vi "ExSpecAppCamera.vi"() -> ()   [LabVIEW 2010]
uses:
  GlobalSpectHdl.vi
  GlobalCamOpen.vi
  GlobalInitializeFlag.vi
  GlobalFramesToStr.vi
  GlobalTimingMode.vi
  GlobalAcquireFocusFlag.vi
  GlobalExposure.vi
  GlobalUserBin.vi
  GlobalCenter.vi
  GlobalFullBin.vi
  GlobalFlipFlag.vi
  GlobalReverseFlag.vi
  GlobalIBackImgHndl.vi
  GlobalIFlatImgHndl.vi
panel:
  out "Spectrometer Active":bool
  in  "Select Spectrometer":bool
  out "Camera Opened":bool
  in  "Exit program":bool
  out "error out":errorcluster
  in  "error in (no error)":errorcluster
  in  "Tab Control":T1(tab)
  in  "Focus/Acquire Mode":u32=1 min=1 max=5 step=1
  in  "Number of Frames to store":u32=1 min=1 step=1
  in  "Intensifier":bool
  in  "Readout Port":i32=-1 min=-1 step=1
  in  "ADC Offset 2":i32=-1 min=-1 step=1
  in  "ADC Gain 2":i32=-1 min=-1 step=1
  in  "ADC speed":i32=-2 min=-3 step=1
  in  "Trigger Edge":u32(ring)=1 items=["N/A", "Positive (leading) edge", "Negative (falling) edge"]
  in  "Timing Mode":u32(ring)=1 items=["N/A", "Free Run/Timed", "Trigger First (PM only)", "Ext Sync/Strobed ", "Variable Exp (PM only)", "Flash Mode (PM only)"]
  out "Pixel Time":i32
  out "Bit Depth":i32
  out "ReadOut port":i32
  out "ADC Offset":i32
  out "ADC Gain":i32
  out "ADC Speed":i32
  in  "Set Experiment \nParameters, Initialize \nCamera/Controller":bool
  out "temperature":dbl format="%.2f"
  out "Temperature Read":dbl(slide) scale=-120.0..20.0
  in  "Temperature":dbl format="%.2f"
  in  "Exposure":dbl format="%.2f"
  out "Controller Initialized":bool
  out "Total":u32
  out "Y dim":u32
  out "X dim":u32
  in  "Y Bin":u32=1 min=1 step=1
  in  "Y Start":u32=1 min=1 step=1
  out "center":bool
  out "User":bool
  out "Full":bool
  in  "Center Strip Button":bool
  in  "User Defined Button":bool
  in  "Full strip Button":bool
  out "Flip\nActive":bool
  in  "Flip flag Button":bool
  out "Reverse\nActive":bool
  in  "Image Reverse Button":bool
  out "Flat Field\nActive":bool
  out "Background \nActive":bool
  in  "Frame number to read":u32=1 min=1 step=1
  in  "Flat Button":bool
  in  "Back Button":bool
  in  "Full File Name":path
  in  "FileType":u32=67371008
  in  "Get Spectrometer \nInformation":bool
  in  "Set Spectrometer":bool
  out "Current Speed":dbl format="%.2f"
  out "Current Gratting":u32
  out "Current Wavelength":dbl format="%.2f"
  in  "Grating number":u32=1 min=1 step=1
  in  "Wavelength":dbl format="%.2f"
  out "Focus graph":sgl[](graph)
  out "Reverse active":bool
  out "Flat Field active":bool
  out "Background active":bool
  in  "Reverse\nbutton":bool
  in  "Flat Field\nbutton":bool
  in  "Background\nbutton":bool
  in  "stop 2":bool
  in  "Start":bool
  out "Camera initialized":bool
  out "Acquire Graph":sgl[](graph)
  out "Collecting Data":bool
  in  "Full File Name for Acqure":path
  in  "OK Button":bool
  out "camera initialized":bool
  # "Note: In order for any parameters to change and be downloaded the initialize button must be hit."
  # "The following are read \nfrom camera after setting\nvalues to left.\n-1 value means item is not \nsupported by camera."
  # "For Slowest ADC speed set this to -3\nFor Fastest ADC speed set this to -2\nTo use current ADC speed don't  hook up or use -1\notherwise put speed in as kHz"
  # "To use current gain don't hook up or set to -1"
  # "To use current gain don't hook up or set to -1"
  # "To use current gain don't hook up or set to -1"
  # "NOTE: if you are using background subtraction or flat field and you change \nthe ROI there are no checks in this example for this."
  # "Pixels coming back\nfrom Camera"
  # "File Types:\nSPE = 67371008\nTIF   = 67174400\nPMI  = 67436544"
  # "Browse match pattern is set to *.tif.  Modify this if different file type is needed."
  # "Note: This is an example only, the user has to verify that the x,y dimensions match for \nthe background and flat field files with the ROI. This error checking logic is not in this \nexample."
  # "Instructions:\nMake sure camera/controller has been initialized, led should be on.\nPress start button, display should appear.\nWhen done press stop button, display should disappear.\nLive buttons only work while collecting data, not before, to setup before goto Live operations tab."
  # "Online operations, will only work while collecting data."
  # "Be sure to put in a full file name below before starting."
  # "Instructions:\nMake sure the camera/controller has been initialized, the light should be on.\nMake sure to put in a file name with path to save data.\nPress Start button and display will pop up and data well be saved in file."
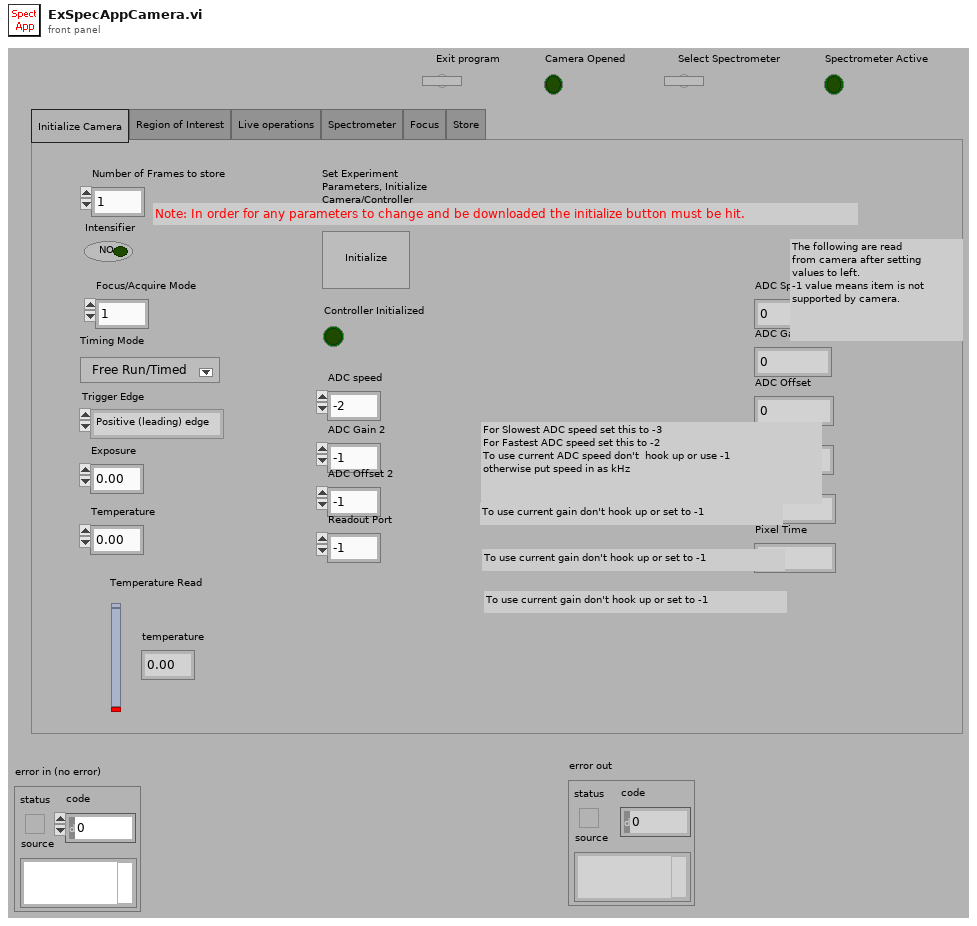
[diagram p1: front panel]
types:
  T1 = enum32{"Initialize Camera", "Region of Interest", "Live operations", "Spectrometer", "Focus", "Store"}
  T2 = cluster{"Camera Handle":u32, "Pulser Handle":u32, "File Handle":u32, "Display Handle":u32, "Image Handle":u32}
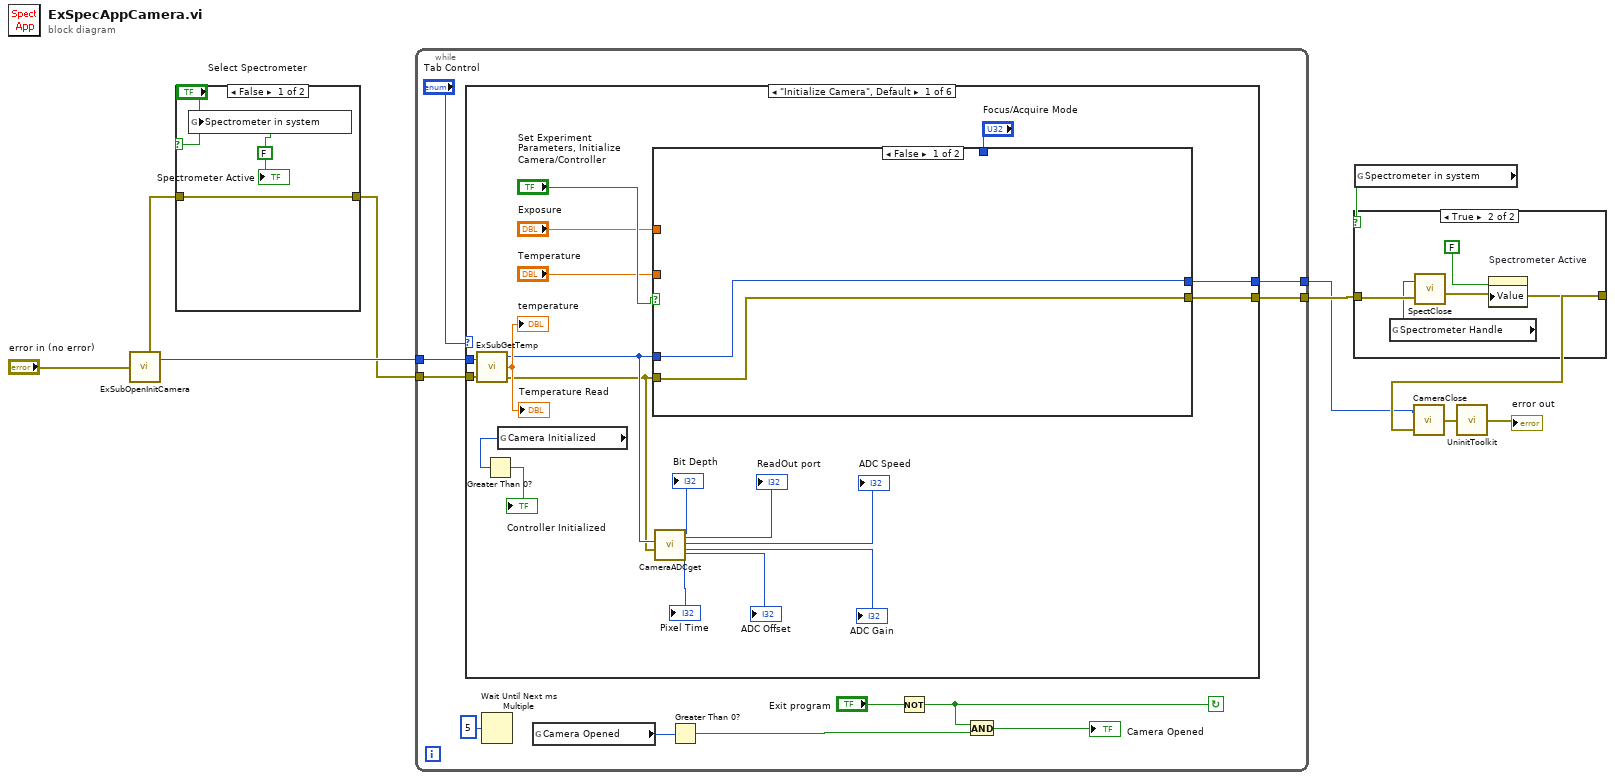
[diagram p0: block diagram]
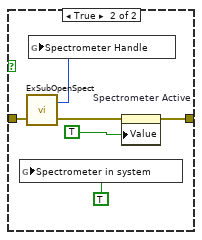
[diagram p3: hidden frame]
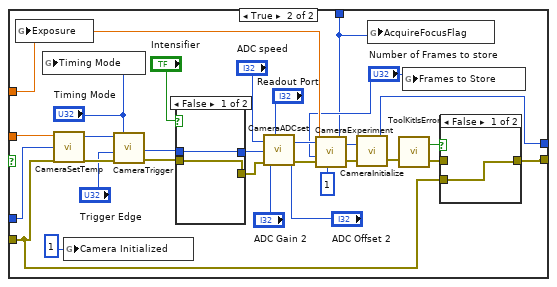
[diagram p4: hidden frame]
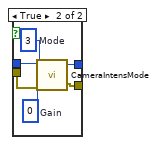
[diagram p6: hidden frame]
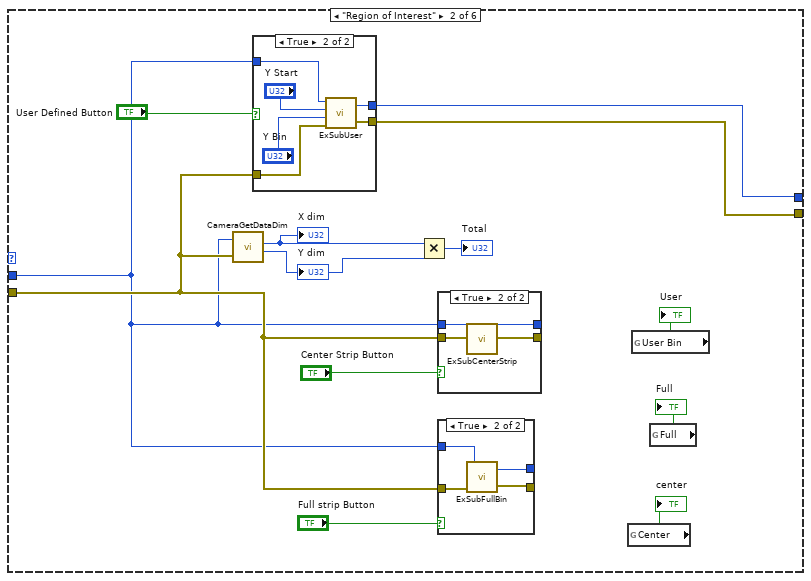
[diagram p7: hidden frame]
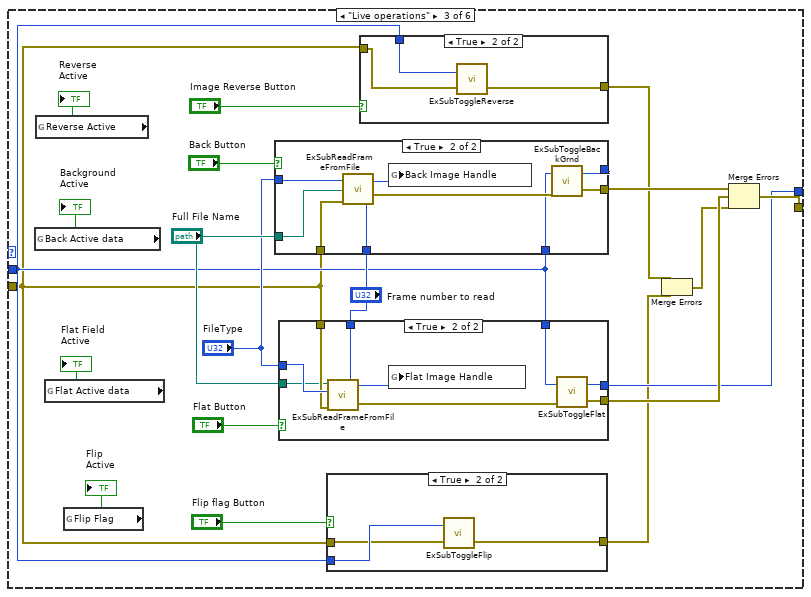
[diagram p11: hidden frame]
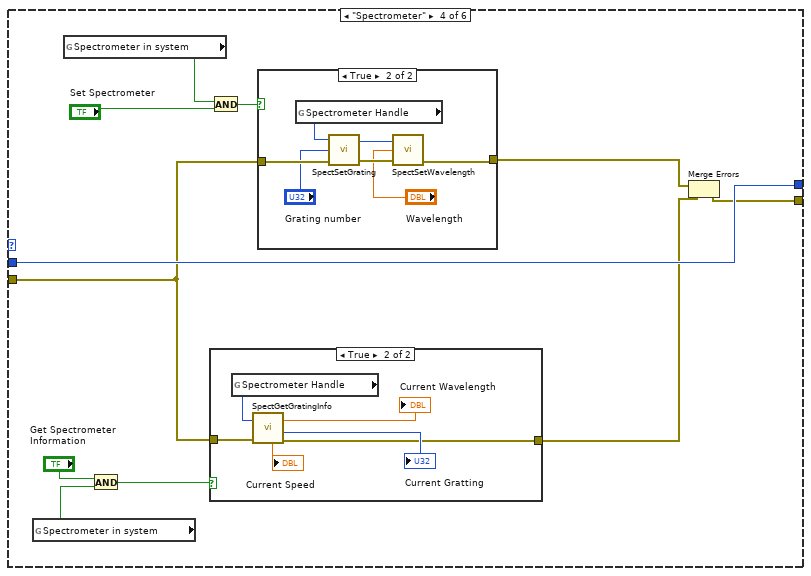
[diagram p16: hidden frame]
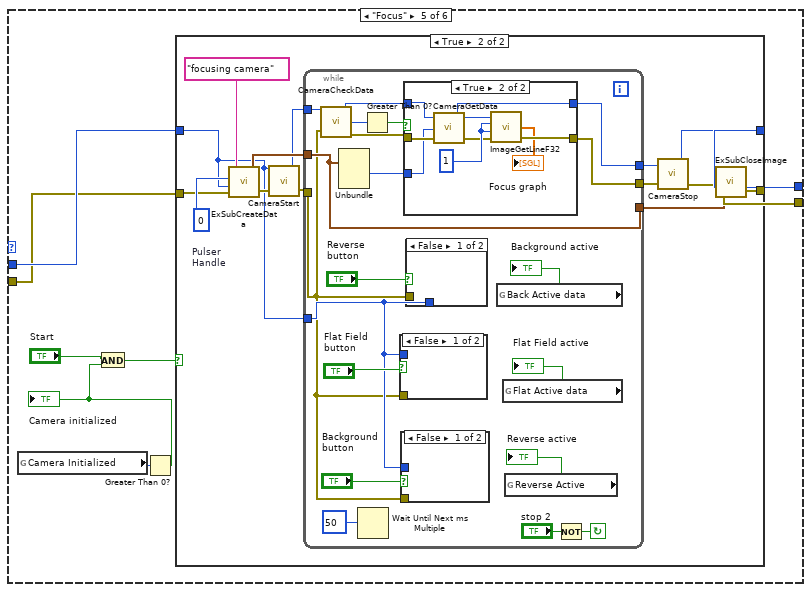
[diagram p19: hidden frame]
diagram:
  n1 = call "ExSubOpenInitCamera.vi"("error in (no error)"="error in (no error)") -> ("Camera Handle"=w2:u32, "error out"=w3:errorcluster)
  n2 = case shown="False" "Select Spectrometer" {
    tunnel: w3 -> [w12 w18]
    tunnel: [w12 w15] -> w1
    frame False {
      w13 = FALSE
      n3 = global write "GlobalSpectHdl.vi" "Spectrometer in system"(w13) -> ()
      "Spectrometer Active" <- w13
    }
    frame True {
      n4 = global write "GlobalSpectHdl.vi" "Spectrometer in system"(TRUE) -> ()
      n5 = call "ExSubOpenSpect.vi"("error in (no error)"=w18) -> ("Spectromete Handle"=w14:u32, "error out"=w17:errorcluster)
      n6 = global write "GlobalSpectHdl.vi" "Spectrometer Handle"(w14) -> ()
      n7 = property on="Spectrometer Active" class="Bool (strict)"(error in=w17, "Value"=TRUE) -> (error out=w15:errorcluster)  [unwired: 1 in, 1 out]
    }
  }
  n8 = while {
    tunnel: w2 -> [w30]
    tunnel: w1 -> [w27]
    tunnel: [w26] -> w6
    tunnel: [w25] -> w8
    stop <- w23 continue-if-true
    n9 = case shown="\"Initialize Camera\", Default" "Tab Control" {
      tunnel: w30 -> [w49 w98 w129 w185 w202 w266]
      tunnel: w27 -> [w41 w99 w128 w178 w201 w265]
      tunnel: [w33 w97 w136 w185 w204 w263] -> w26
      tunnel: [w32 w96 w137 w177 w203 w264] -> w25
      frame "Initialize Camera", Default {
        n10 = call "ExSubGetTemp.vi"("Camera Handle"=w49, "error in (no error)"=w41) -> ("Camera Handle"=w40:u32, "Temperature Real"=→"temperature" →"Temperature Read":dbl, "error out"=w39:errorcluster)
        n11 = global read "GlobalInitializeFlag.vi" "Camera Initialized"() -> (w44:u32)
        n12 = Greater Than 0?(x=w44) -> (x > 0?=→"Controller Initialized":bool)
        n13 = case shown="False" "Set Experiment \nParameters, Initialize \nCamera/Controller" {
          tunnel: "Exposure" -> [_ w70]
          tunnel: "Temperature" -> [_ w79]
          tunnel: w39 -> [w50 w54]
          tunnel: w40 -> [w51 w80]
          tunnel: [w50 w57] -> w32
          tunnel: [w51 w55] -> w33
          tunnel: "Focus/Acquire Mode" -> [_ w52]
          frame False {
          }
          frame True {
            n14 = global write "GlobalExposure.vi" "Exposure"(w70) -> ()
            n15 = global write "GlobalTimingMode.vi" "Timing Mode"("Timing Mode") -> ()
            n16 = call <userlib>:"CameraSetTemp.vi"("error in (no error)"=w54, "Temperature"=w79, "Camera Handle"=w80) -> ("error out"=w69:errorcluster, "Camera Handle"=w68:u32)
            n17 = global write "GlobalInitializeFlag.vi" "Camera Initialized"(1) -> ()
            n18 = call <userlib>:"CameraTrigger.vi"("error in"=w69, "Trigger Edge"="Trigger Edge", "Timing Mode"="Timing Mode", "Camera Handle"=w68) -> ("error out"=w65:errorcluster, "Camera Handle"=w66:u32)
            n19 = case shown="False" "Intensifier" {
              tunnel: [w85 w91] -> w76
              tunnel: [w84 w90] -> w77
              tunnel: w66 -> [w85 w87]
              tunnel: w65 -> [w84 w86]
              frame False {
              }
              frame True {
                w88 = u32 0  # Gain
                w89 = u32 3  # Mode
                n20 = call <userlib>:"CameraIntensMode.vi"("error in"=w86, "Intensifier Gain"=w88, "Mode"=w89, "Camera Handle"=w87) -> ("error out"=w90:errorcluster, "Camera Handle"=w91:u32)
              }
            }
            n21 = call <userlib>:"CameraADCset.vi"("ADC offset"="ADC Offset 2", "Read Out port"="Readout Port", "error in (no error)"=w77, "ADC Gain"="ADC Gain 2", "ADC Speed"="ADC speed", "Camera Handle"=w76) -> ("error out"=w63:errorcluster, "Camera Handle"=w62:u32)
            n22 = call <userlib>:"CameraExperiment.vi"("Number of Accumulations"=1, "Acquire / Focus Flag"=w52, "error in"=w63, "Number of Images"="Number of Frames to store", "Exposure (sec)"=w70, "Camera Handle"=w62) -> ("error out"=w61:errorcluster, "Camera Handle"=w60:u32)
            n23 = call <userlib>:"CameraInitialize.vi"("error in"=w61, "Camera Handle"=w60) -> ("error out"=w56:errorcluster, "Camera Handle"=w55:u32)
            n24 = global write "GlobalAcquireFocusFlag.vi" "AcquireFocusFlag"(w52) -> ()
            n25 = call <userlib>:"ToolKitIsError.vi"("error in"=w56) -> ("error out"=w58:errorcluster, "Error Flag"=w59:bool)  [unwired: 1 in]
            n26 = global write "GlobalFramesToStr.vi" "Frames to Store"("Number of Frames to store") -> ()
            n27 = case shown="False" w59 {
              tunnel: w58 -> [_ w83]
              tunnel: [w82 w83] -> w57
              tunnel: w54 -> [w82 _]
              frame False {
              }
              frame True {
              }
            }
          }
        }
        n28 = call <userlib>:"CameraADCget.vi"("Camera handle"=w40, "error in (no error)"=w39) -> ("Bit Depth"=→"Bit Depth":i32, "Pixel Time"=→"Pixel Time":i32, "Readout Port"=→"ReadOut port":i32, "ADC Offset"=→"ADC Offset":i32, "ADC Speed"=→"ADC Speed":i32, "ADC Gain"=→"ADC Gain":i32)  [unwired: 2 out]
      }
      frame "Region of Interest" {
        n29 = call <userlib>:"CameraGetDataDim.vi"("Camera Handle"=w98, "error in"=w99) -> ("Xdim"=w95:u32, "Ydim"=w94:u32)  [unwired: 2 out]
        "X dim" <- w95
        "Y dim" <- w94
        n30 = case shown="True" "User Defined Button" {
          tunnel: w98 -> [w117 w124]
          tunnel: [w117 w119] -> w97
          tunnel: w99 -> [w118 w121]
          tunnel: [w118 w120] -> w96
          frame False {
          }
          frame True {
            n31 = call "ExSubUser.vi"("error in (no error)"=w121, "Y Bin"="Y Bin", "Y Start"="Y Start", "Camera Handle"=w124) -> ("error out"=w120:errorcluster, "Camera Handle"=w119:u32)
          }
        }
        n32 = Multiply(x=w95, y=w94) -> (x*y=→"Total":u32)
        n33 = case shown="True" "Center Strip Button" {
          tunnel: w98 -> [w112 w115]
          tunnel: [w112 w114] -> _
          tunnel: w99 -> [w111 w116]
          tunnel: [w111 w113] -> _
          frame False {
          }
          frame True {
            n34 = call "ExSubCenterStrip.vi"("error in (no error)"=w116, "Camera Handle"=w115) -> ("error out"=w113:errorcluster, "Camera Handle"=w114:u32)
          }
        }
        n35 = case shown="True" "Full strip Button" {
          tunnel: w98 -> [w106 w110]
          tunnel: [w106 w108] -> _
          tunnel: w99 -> [w105 w109]
          tunnel: [w105 w107] -> _
          frame False {
          }
          frame True {
            n36 = call "ExSubFullBin.vi"("error in (no error)"=w109, "Camera Handle"=w110) -> ("error out"=w107:errorcluster, "Camera Handle"=w108:u32)
          }
        }
        n37 = global read "GlobalCenter.vi" "Center"() -> (→"center":bool)
        n38 = global read "GlobalUserBin.vi" "User Bin"() -> (→"User":bool)
        n39 = global read "GlobalFullBin.vi" "Full"() -> (→"Full":bool)
      }
      frame "Live operations" {
        n40 = global read "GlobalIBackImgHndl.vi" "Back Active data"() -> (→"Background \nActive":bool)
        n41 = global read "GlobalReverseFlag.vi" "Reverse Active"() -> (→"Reverse\nActive":bool)
        n42 = global read "GlobalIFlatImgHndl.vi" "Flat Active data"() -> (→"Flat Field\nActive":bool)
        n43 = global read "GlobalFlipFlag.vi" "Flip Flag"() -> (→"Flip\nActive":bool)
        n44 = case shown="True" "Back Button" {
          tunnel: "Full File Name" -> [_ w172]
          tunnel: "FileType" -> [_ w173]
          tunnel: w128 -> [w165 w174]
          tunnel: [w165 w168] -> w139
          tunnel: "Frame number to read" -> [_ w171]
          tunnel: w129 -> [w164 w167]
          tunnel: [w164 w166] -> _
          frame False {
          }
          frame True {
            n45 = call "ExSubReadFrameFromFile.vi"("error in (no error)"=w174, "Frame to pull off"=w171, "File type"=w173, "path to file to open"=w172) -> ("error out"=w169:errorcluster, "Image Handle"=w170:u32)
            n46 = global write "GlobalIBackImgHndl.vi" "Back Image Handle"(w170) -> ()
            n47 = call "ExSubToggleBackGrnd.vi"("error in (no error)"=w169, "Camera Handle"=w167) -> ("error out"=w168:errorcluster, "Camera Handle"=w166:u32)
          }
        }
        n48 = case shown="True" "Flat Button" {
          tunnel: "Full File Name" -> [_ w160]
          tunnel: "FileType" -> [_ w163]
          tunnel: w128 -> [w154 w161]
          tunnel: [w154 w156] -> w138
          tunnel: "Frame number to read" -> [_ w162]
          tunnel: w129 -> [w153 w158]
          tunnel: [w153 w157] -> w136
          frame False {
          }
          frame True {
            n49 = call "ExSubReadFrameFromFile.vi"("error in (no error)"=w161, "Frame to pull off"=w162, "File type"=w163, "path to file to open"=w160) -> ("error out"=w155:errorcluster, "Image Handle"=w159:u32)
            n50 = global write "GlobalIFlatImgHndl.vi" "Flat Image Handle"(w159) -> ()
            n51 = call "ExSubToggleFlat.vi"("error in (no error)"=w155, "Camera Handle"=w158) -> ("error out"=w156:errorcluster, "Camera Handle"=w157:u32)
          }
        }
        n52 = case shown="True" "Flip flag Button" {
          tunnel: w129 -> [_ w152]
          tunnel: w128 -> [w149 w151]
          tunnel: [w149 w150] -> w127
          frame False {
          }
          frame True {
            n53 = call "ExSubToggleFlip.vi"("error in (no error)"=w151, "Camera Handle"=w152) -> ("error out"=w150:errorcluster)  [unwired: 1 out]
          }
        }
        n54 = case shown="True" "Image Reverse Button" {
          tunnel: w129 -> [_ w147]
          tunnel: w128 -> [w145 w148]
          tunnel: [w145 w146] -> w126
          frame False {
          }
          frame True {
            n55 = call "ExSubToggleReverse.vi"("error in (no error)"=w148, "Camera Handle"=w147) -> ("error out"=w146:errorcluster)  [unwired: 1 out]
          }
        }
        n56 = Merge Errors(w126, w127) -> (w125:errorcluster)
        n57 = Merge Errors(w139, w138, w125) -> (w137:errorcluster)
      }
      frame "Spectrometer" {
        n58 = global read "GlobalSpectHdl.vi" "Spectrometer in system"() -> (w181:bool)
        n59 = global read "GlobalSpectHdl.vi" "Spectrometer in system"() -> (w184:bool)
        n60 = And(x="Get Spectrometer \nInformation", y=w181) -> (x .and. y?=w179:bool)
        n61 = case shown="True" w179 {
          tunnel: w178 -> [w186 w191]
          tunnel: [w186 w188] -> w176
          frame False {
          }
          frame True {
            n62 = global read "GlobalSpectHdl.vi" "Spectrometer Handle"() -> (w192:u32)
            n63 = call <userlib>:"SpectGetGratingInfo.vi"("Spectrometer Handle"=w192, "error in"=w191) -> ("Current Wavelength"=→"Current Wavelength":dbl, "Current Speed"=→"Current Speed":dbl, "Current Grating"=→"Current Gratting":i16, "error out"=w188:errorcluster)  [unwired: 2 out]
          }
        }
        n64 = And(x=w184, y="Set Spectrometer") -> (x .and. y?=w182:bool)
        n65 = case shown="True" w182 {
          tunnel: w178 -> [w193 w199]
          tunnel: [w193 w194] -> w175
          frame False {
          }
          frame True {
            n66 = global read "GlobalSpectHdl.vi" "Spectrometer Handle"() -> (w200:u32)
            n67 = call <userlib>:"SpectSetGrating.vi"("error in"=w199, "Grating Number"="Grating number", "Sepctrometer Handle"=w200) -> ("error out"=w196:errorcluster, "Spectrometer Handle"=w197:u32)
            n68 = call <userlib>:"SpectSetWavelength.vi"("error in"=w196, "Wavelength"="Wavelength", "Spectrometer Handle"=w197) -> ("error out"=w194:errorcluster)  [unwired: 1 out]
          }
        }
        n69 = Merge Errors(w175, w176) -> (w177:errorcluster)
      }
      frame "Focus" {
        n70 = global read "GlobalInitializeFlag.vi" "Camera Initialized"() -> (w206:u32)
        n71 = Greater Than 0?(x=w206) -> (x > 0?=w205:bool)
        "Camera initialized" <- w205
        n72 = And(x="Start", y=w205) -> (x .and. y?=w208:bool)
        n73 = case shown="True" w208 {
          tunnel: w201 -> [w209 w220]
          tunnel: w202 -> [w210 w213]
          tunnel: [w210 w218] -> w204
          tunnel: [w209 w217] -> w203
          frame False {
          }
          frame True {
            w221 = u32 0  # Pulser  Handle
            n74 = call "ExSubCreateData.vi"("error in (no error)"=w220, "File and Display Name"="focusing camera", "Pulser Handle"=w221, "Camera Handle"=w213) -> ("error out"=w222:errorcluster, "Handles Out"=w224:T2)
            n75 = call <userlib>:"CameraStart.vi"("error in"=w222, "Camera Handle"=w213) -> ("error out"=w223:errorcluster, "Camera Handle"=w215:u32)
            n76 = while {
              tunnel: w224 -> [w226]
              tunnel: w223 -> [w225]
              tunnel: w213 -> [w238]
              tunnel: w215 -> [w230]
              tunnel: [w229] -> w214
              tunnel: [w228] -> w212
              tunnel: [w226] -> w211
              stop <- w242 continue-if-true
              n77 = call <userlib>:"CameraCheckData.vi"("Camera Handle"=w230, "error in"=w225) -> ("Camera Handle"=w232:u32, "Number Of Frames Available"=w234:i32, "error out"=w231:errorcluster)
              n78 = Unbundle(w226) -> ("Image Handle"=w227:u32)  [unwired: 4 out]
              n79 = Wait Until Next ms Multiple(millisecond multiple=u32 50) -> ()  [unwired: 1 out]
              n80 = Greater Than 0?(x=w234) -> (x > 0?=w233:bool)
              n81 = case shown="False" "Flat Field\nbutton" {
                tunnel: w238 -> [_ w258]
                tunnel: w225 -> [_ w259]
                frame False {
                }
                frame True {
                  n82 = call "ExSubToggleFlat.vi"("error in (no error)"=w259, "Camera Handle"=w258) -> ()  [unwired: 2 out]
                }
              }
              n83 = case shown="False" "Background\nbutton" {
                tunnel: w238 -> [_ w257]
                tunnel: w225 -> [_ w256]
                frame False {
                }
                frame True {
                  n84 = call "ExSubToggleBackGrnd.vi"("error in (no error)"=w256, "Camera Handle"=w257) -> ()  [unwired: 2 out]
                }
              }
              n85 = case shown="True" w233 {
                tunnel: w232 -> [w246 w255]
                tunnel: w231 -> [w245 w254]
                tunnel: [w245 w249] -> w228
                tunnel: [w246 w248] -> w229
                tunnel: w227 -> [_ w253]
                frame False {
                }
                frame True {
                  w251 = 1
                  n86 = call <userlib>:"CameraGetData.vi"("error in"=w254, "Data Handle"=w253, "Camera Handle"=w255) -> ("error out"=w250:errorcluster, "Data Handle"=w252:u32, "Camera Handle"=w248:u32)
                  n87 = call <userlib>:"ImageGetLineF32.vi"("error in"=w250, "Z Position"=w251, "Y Position"=w251, "Data Handle"=w252) -> ("error out"=w249:errorcluster, "Array F32"=→"Focus graph":sgl[])  [unwired: 1 out]
                }
              }
              n88 = case shown="False" "Reverse\nbutton" {
                tunnel: w225 -> [_ w261]
                tunnel: w238 -> [_ w260]
                frame False {
                }
                frame True {
                  n89 = call "ExSubToggleReverse.vi"("error in (no error)"=w261, "Camera Handle"=w260) -> ()  [unwired: 2 out]
                }
              }
              n90 = global read "GlobalIBackImgHndl.vi" "Back Active data"() -> (→"Background active":bool)
              n91 = global read "GlobalIFlatImgHndl.vi" "Flat Active data"() -> (→"Flat Field active":bool)
              n92 = global read "GlobalReverseFlag.vi" "Reverse Active"() -> (→"Reverse active":bool)
              n93 = Not(x="stop 2") -> (.not. x?=w242:bool)
            }
            n94 = call <userlib>:"CameraStop.vi"("error in"=w212, "Camera Handle"=w214) -> ("error out"=w219:errorcluster, "Camera Handle"=w218:u32)
            n95 = call "ExSubCloseImage.vi"("error in (no error)"=w219, "Handles In"=w211) -> ("error out"=w217:errorcluster)
          }
        }
      }
      frame "Store" {
        n96 = global read "GlobalInitializeFlag.vi" "Camera Initialized"() -> (w268:u32)
        n97 = Greater Than 0?(x=w268) -> (x > 0?=w267:bool)
        "camera initialized" <- w267
        n98 = And(x="OK Button", y=w267) -> (x .and. y?=w270:bool)
        n99 = case shown="True" w270 {
          tunnel: w266 -> [w272 w278]
          tunnel: w265 -> [w271 w282]
          tunnel: [w271 w283] -> w264
          tunnel: [w272 w279] -> w263
          frame False {
          }
          frame True {
            w289 = u32 0  # Pulser Handle
            n100 = global read "GlobalFramesToStr.vi" "Frames to Store"() -> (w285:u32)
            n101 = property on="Collecting Data" class="Bool (strict)"(error in=w282, "Value"=TRUE) -> (error out=w281:errorcluster)  [unwired: 1 in, 1 out]
            n102 = Path To String(path="Full File Name for Acqure") -> (string=w287:string)
            n103 = call "ExSubCreateFile.vi"("error in (no error)"=w281, "File and Display Name"=w287, "Pulser Handle"=w289, "Camera Handle"=w278) -> ("error out"=w290:errorcluster, "Handles Out"=w275:T2)
            n104 = Unbundle(w275) -> ("File Handle"=w276:u32, "Image Handle"=w273:u32)  [unwired: 3 out]
            n105 = call <userlib>:"CameraStart.vi"("error in"=w290, "Camera Handle"=w278) -> ("error out"=w274:errorcluster, "Camera Handle"=w284:u32)
            n106 = for {
              N: w285 -> [_]
              tunnel: w278 -> [w295]
              tunnel: w274 -> [w294]
              tunnel: [w293] -> w277
              tunnel: w276 -> [w292]
              tunnel: w273 -> [w291]
              n107 = while {
                tunnel: [w302] -> w293
                tunnel: w295 -> [w300]
                tunnel: w294 -> [w299]
                tunnel: w292 -> [w298]
                tunnel: w291 -> [w297]
                stop <- w303 stop-if-true
                n108 = call <userlib>:"CameraCheckData.vi"("Camera Handle"=w300, "error in"=w299) -> ("Camera Handle"=w305:u32, "Number Of Frames Available"=w307:i32, "error out"=w304:errorcluster)
                n109 = Greater Than 0?(x=w307) -> (x > 0?=w306:bool)
                n110 = case shown="True" w306 {
                  selector: w306 -> [w308 w318]
                  tunnel: w305 -> [_ w320]
                  tunnel: w304 -> [w309 w319]
                  tunnel: [w308 w318] -> w303
                  tunnel: [w309 w313] -> w302
                  tunnel: w298 -> [_ w311]
                  tunnel: w297 -> [_ w310]
                  frame False {
                  }
                  frame True {
                    w314 = 1
                    n111 = call <userlib>:"CameraGetData.vi"("error in"=w319, "Data Handle"=w310, "Camera Handle"=w320) -> ("error out"=w317:errorcluster, "Data Handle"=w315:u32)  [unwired: 1 out]
                    n112 = call <userlib>:"FileSaveData.vi"("error in"=w317, "Image Handle"=w315, "File Handle"=w311) -> ("error out"=w316:errorcluster)  [unwired: 1 out]
                    n113 = call <userlib>:"ImageGetLineF32.vi"("error in"=w316, "Z Position"=w314, "Y Position"=w314, "Data Handle"=w315) -> ("error out"=w313:errorcluster, "Array F32"=→"Acquire Graph":sgl[])  [unwired: 1 out]
                  }
                }
                n114 = Wait Until Next ms Multiple(millisecond multiple=u32 50) -> ()  [unwired: 1 out]
              }
              n115 = Wait Until Next ms Multiple(millisecond multiple=u32 50) -> ()  [unwired: 1 out]
            }
            n116 = call <userlib>:"CameraStop.vi"("error in"=w277, "Camera Handle"=w284) -> ("error out"=w286:errorcluster, "Camera Handle"=w279:u32)
            n117 = call "ExSubCloseFileImage.vi"("error in (no error)"=w286, "Handles In"=w275) -> ("error out"=w283:errorcluster)
          }
        }
        "Collecting Data" <- FALSE
      }
    }
    n118 = Wait Until Next ms Multiple(millisecond multiple=5) -> ()  [unwired: 1 out]
    n119 = global read "GlobalCamOpen.vi" "Camera Opened"() -> (w24:u32)
    n120 = Greater Than 0?(x=w24) -> (x > 0?=w22:bool)
    n121 = Not(x="Exit program") -> (.not. x?=w23:bool)
    n122 = And(x=w23, y=w22) -> (x .and. y?=→"Camera Opened":bool)
  }
  n123 = global read "GlobalSpectHdl.vi" "Spectrometer in system"() -> (w5:bool)
  n124 = case shown="True" w5 {
    tunnel: w8 -> [w321 w326]
    tunnel: [w321 w324] -> w7
    frame False {
    }
    frame True {
      n125 = global read "GlobalSpectHdl.vi" "Spectrometer Handle"() -> (w322:u32)
      n126 = call <userlib>:"SpectClose.vi"("error in"=w326, "Spectrometer Handle"=w322) -> ("error out"=w325:errorcluster)
      n127 = property on="Spectrometer Active" class="Bool (strict)"(error in=w325, "Value"=FALSE) -> (error out=w324:errorcluster)  [unwired: 1 in, 1 out]
    }
  }
  n128 = call <userlib>:"CameraClose.vi"("error in"=w7, "Camera Handle"=w6) -> ("error out"=w11:errorcluster)
  n129 = call <userlib>:"UninitToolkit.vi"("error in"=w11) -> ("error out"=→"error out":errorcluster)
